vi "Correct Flow Rate and Get Dilution Factors.vi"(7 "Qbank":sgl, 8 "error in":errorcluster, 9 "RHbank":sgl, 10 "Qpurge":sgl, 11 "CRDS Cell in":refnum<class "CRDS Cell.lvclass">) -> (0 "error out":errorcluster, 3 "CRDS Cell out":refnum<class "CRDS Cell.lvclass">)   [LabVIEW 2015, in "CRDS Cell.lvclass"]
doc: "Calculate the cell relative properties. RH and flow rates will be measured only one time for each cell bank and therefore we need to account for dilution. In addition, the extinction will be affected by the purge flows and must be accounted for in each cell. \n\nBoth the RH and flow rates are based on the relative volume of air associated with the bulk and purge flows and therefore have the same dilution factor. The assumption is that the RH in a particular cell will be affected only by the upstream purge flows. This assumption is correct given that diffusion is slow relative to the length of the cells."
uses:
  CRDS Cell.lvclass
  CRDS Cell.lvclass/CRDS Cell.ctl
  Data/Cell/Read hkParam.vi
  Data/Cell/Write hkParam.vi
  Data/Cell/CRDS Cell Data.lvclass
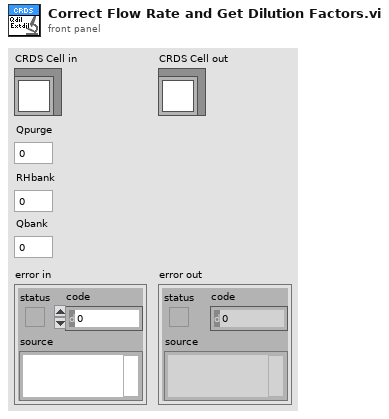
[diagram p1: front panel]
types:
  T1 = typedef "Base CRDS Lib.lvlib/calData.ctl" = cluster{"rhDilFac":sgl, "Q":sgl, "Tmean":sgl, "extDilFac":sgl, "rhCell":sgl, "P":sgl, "T":sgl}
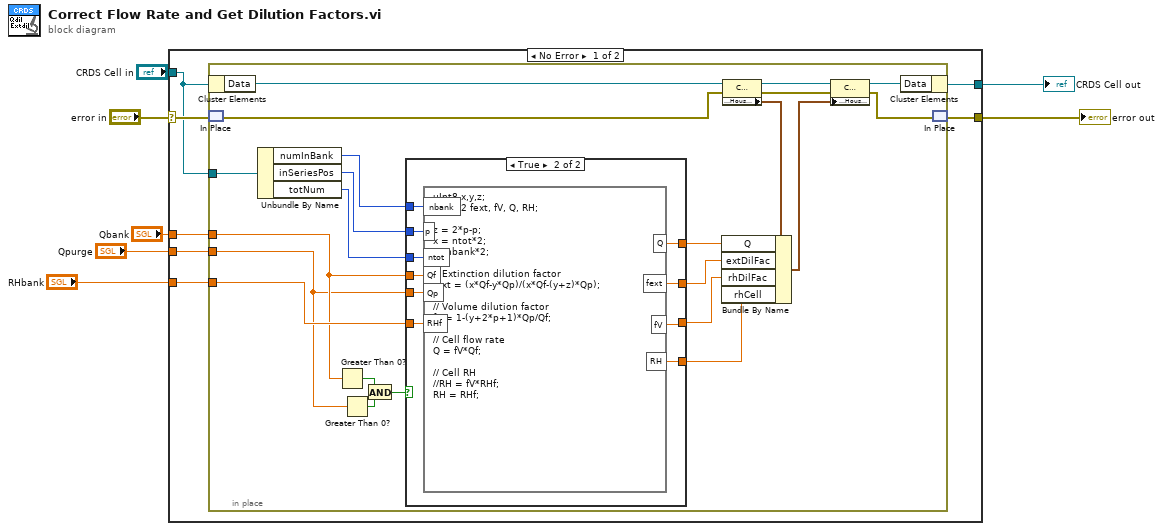
[diagram p0: block diagram]
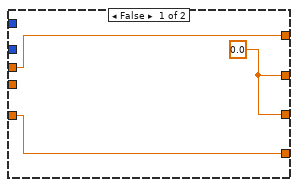
[diagram p2: hidden frame]
diagram:
  n1 = case shown="No Error" "error in" {
    selector: "error in" -> [w10 w51]
    tunnel: [w9 w51] -> w6
    tunnel: [w11 w50] -> w4
    tunnel: "CRDS Cell in" -> [w8 w50]
    tunnel: "Qpurge" -> [w12 _]
    tunnel: "Qbank" -> [w13 _]
    tunnel: "RHbank" -> [w14 _]
    frame No Error {
      n2 = in-place {
        in-place-border: w14 -> [w25]
        in-place-border: w13 -> [w24]
        in-place-border: w12 -> [w23]
        in-place-border: w8 -> [w15]
        n3 = in-place-cluster #1(w8) -> ("Data"=w19:refnum<class "CRDS Cell Data.lvclass">)
        n4 = in-place-match #2(w10) -> (w17:errorcluster)
        n5 = Unbundle By Name(w15) -> ("numInBank"=w31:u8, "inSeriesPos"=w30:u8, "totNum"=w32:u8)
        n6 = Greater Than 0?(x=w24) -> (x > 0?=w21:bool)
        n7 = Greater Than 0?(x=w23) -> (x > 0?=w22:bool)
        n8 = And(x=w21, y=w22) -> (x .and. y?=w20:bool)
        n9 = case shown="True" w20 {
          tunnel: w32 -> [_ w49]
          tunnel: w24 -> [w39 w48]
          tunnel: w31 -> [_ w47]
          tunnel: w30 -> [_ w46]
          tunnel: [w38 w45] -> w29
          tunnel: [w38 w44] -> w28
          tunnel: [w39 w43] -> w27
          tunnel: w23 -> [_ w42]
          tunnel: [w37 w41] -> w26
          tunnel: w25 -> [w37 w40]
          frame False {
            w38 = sgl 0.0
          }
          frame True {
            n10 = formula code="uInt8 x,y,z;\nfloat32 fext, fV, Q, RH;\n\nz = 2*p-p;\nx = ntot*2;\ny=nbank*2;\n\n// Extinction dilution factor\nfext = (x*Qf-y*Qp)/(x*Qf-(y+z)*Qp);\n\n// Volume dilution factor\nfV = 1-(y+2*p+1)*Qp/Qf;\n\n// Cell flow rate\nQ = fV*Qf;\n\n// Cell RH\n//RH = fV*RHf;\nRH = RHf;"("nbank"=w47, "p"=w46, "ntot"=w49, "Qf"=w48, "Qp"=w42, "RHf"=w40) -> ("fext"=w45:sgl, "fV"=w44:sgl, "Q"=w43:sgl, "RH"=w41:sgl)
          }
        }
        n11 = property class="CRDS Cell"(reference=w19, error in=w17) -> (reference out=w35:refnum<class "CRDS Cell Data.lvclass">, error out=w33:errorcluster, "Data Access:Housekeeping"=w36:T1)
        n12 = Bundle By Name(cluster=w36, "Q"=w27, "extDilFac"=w29, "rhDilFac"=w28, "rhCell"=w26) -> (w34:T1)
        n13 = property class="CRDS Cell"(reference=w35, error in=w33, "Data Access:Housekeeping"=w34) -> (reference out=w18:refnum<class "CRDS Cell Data.lvclass">, error out=w16:errorcluster)
        n14 = in-place-cluster #1("Data"=w18) -> (w11:refnum<class "CRDS Cell.lvclass">)
        n15 = in-place-match #2(w16) -> (w9:errorcluster)
      }
    }
    frame Error {
    }
  }
  "error out" <- w6
  "CRDS Cell out" <- w4
